vi "price.vi"(8 "error in (no error)":errorcluster, 11 "Burger in":refnum<class "Burger.lvclass">) -> (0 "error out":errorcluster, 2 "price":dbl, 3 "Burger out":refnum<class "Burger.lvclass">)   [LabVIEW 2017, in "Burger.lvclass"]
uses:
  Burger.lvclass
  Item Class/Item.lvclass
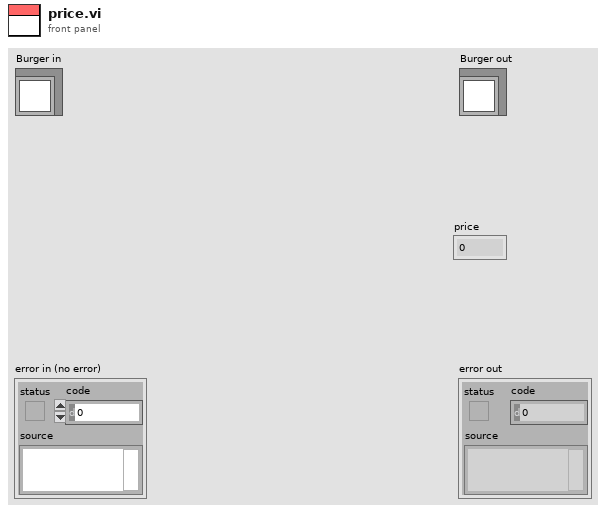
[diagram p1: front panel]
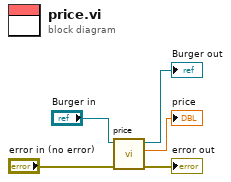
[diagram p0: block diagram]
diagram:
  n1 = call-parent "price.vi"("error in (no error)"="error in (no error)", "Item in"="Burger in") -> ("error out"=→"error out":errorcluster, "price"=→"price":dbl, "Item out"=→"Burger out":refnum<class "Burger.lvclass">)  [unwired: 7 in]
